vi "getSFP+ResultCluster.vi"(9 "itemClusters":T2) -> (3 "resultCluster":T1)   [LabVIEW 2011]
panel:
  in  "resultCluster":T1
  out "TDD":string
  out "NEXT":string
  out "SCC11":string
  out "SCD21-SDD21":string
  out "ILD":string
  out "SDD11":string
  out "SDD21":string
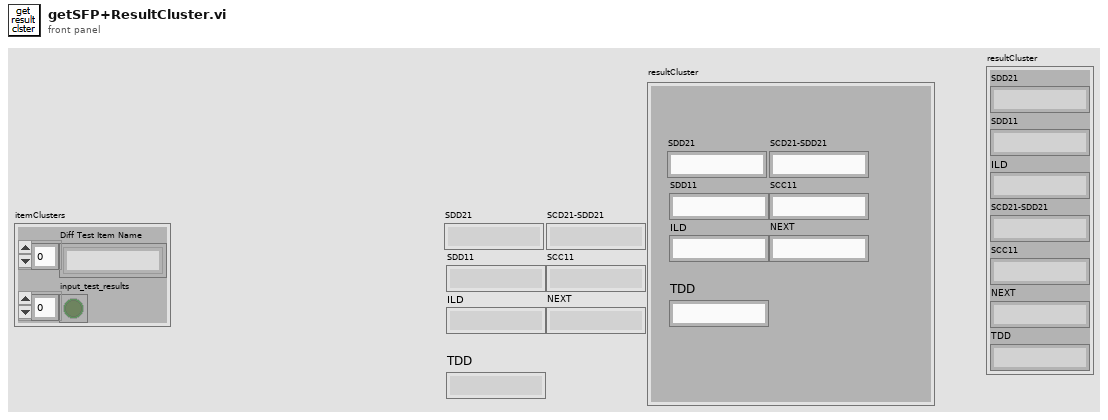
[diagram p1: front panel]
types:
  T1 = cluster{"SDD21":string, "SDD11":string, "ILD":string, "SCD21-SDD21":string, "SCC11":string, "NEXT":string, "TDD":string}
  T2 = cluster{"Diff Test Item Name":string[], "input_test_results":bool[]}
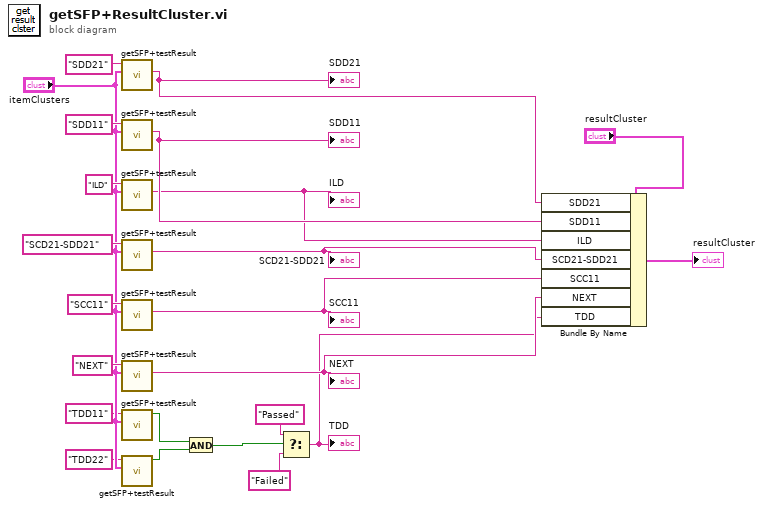
[diagram p0: block diagram]
diagram:
  n1 = call "getSFP+testResult.vi"("itemClusters"="itemClusters", "itemName"="SDD21") -> ("sResult"=w9:string)  [unwired: 8 in, 1 out]
  "SDD21" <- w9
  n2 = call "getSFP+testResult.vi"("itemClusters"="itemClusters", "itemName"="SDD11") -> ("sResult"=w7:string)  [unwired: 8 in, 1 out]
  "SDD11" <- w7
  n3 = call "getSFP+testResult.vi"("itemClusters"="itemClusters", "itemName"="ILD") -> ("sResult"=w6:string)  [unwired: 8 in, 1 out]
  "ILD" <- w6
  n4 = call "getSFP+testResult.vi"("itemClusters"="itemClusters", "itemName"="SCD21-SDD21") -> ("sResult"=w5:string)  [unwired: 8 in, 1 out]
  "SCD21-SDD21" <- w5
  n5 = call "getSFP+testResult.vi"("itemClusters"="itemClusters", "itemName"="SCC11") -> ("sResult"=w4:string)  [unwired: 8 in, 1 out]
  "SCC11" <- w4
  n6 = call "getSFP+testResult.vi"("itemClusters"="itemClusters", "itemName"="NEXT") -> ("sResult"=w3:string)  [unwired: 8 in, 1 out]
  "NEXT" <- w3
  n7 = call "getSFP+testResult.vi"("itemClusters"="itemClusters", "itemName"="TDD11") -> ("result"=w14:bool)  [unwired: 8 in, 1 out]
  n8 = call "getSFP+testResult.vi"("itemClusters"="itemClusters", "itemName"="TDD22") -> ("result"=w13:bool)  [unwired: 8 in, 1 out]
  n9 = And(x=w14, y=w13) -> (x .and. y?=w10:bool)
  n10 = Select(t="Passed", s=w10, f="Failed") -> (s? t:f=w2:string)
  "TDD" <- w2
  n11 = Bundle By Name(cluster="resultCluster", "SDD21"=w9, "SDD11"=w7, "ILD"=w6, "SCD21-SDD21"=w5, "SCC11"=w4, "NEXT"=w3, "TDD"=w2) -> (→"resultCluster":T1)
